vi "Number manipulating.vi"() -> ()   [LabVIEW 2017]
panel:
  in  "y 2":dbl
  in  "y":dbl
  out "x/y 2":dbl
  out "x/y":dbl
  in  "Numeric":i32
  out "Array":string[](array[string])
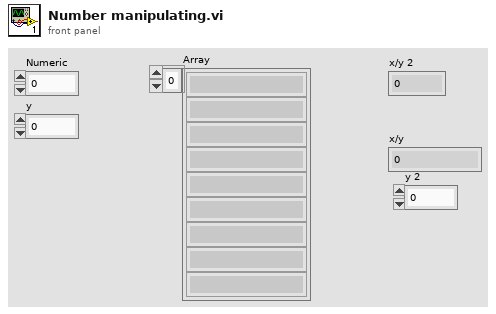
[diagram p1: front panel]
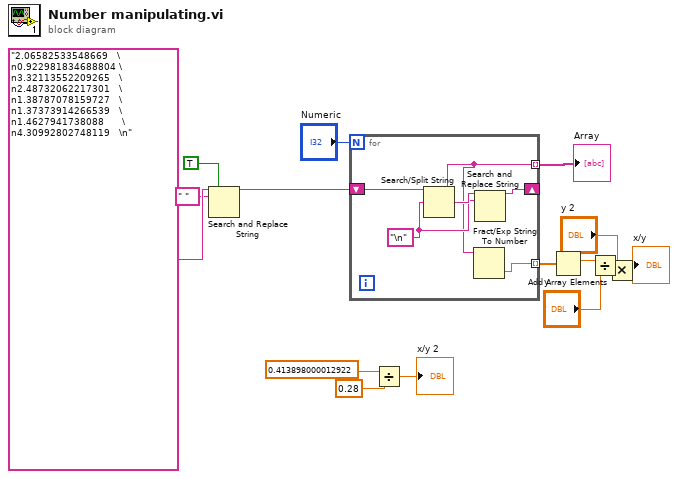
[diagram p0: block diagram]
diagram:
  n1 = Search and Replace String(replace all?=TRUE ("replace all? (F)"), input string="2.06582533548669   \n0.922981834688804 \n3.32113552209265   \n2.48732062217301   \n1.38787078159727   \n1.37373914266539   \n1.4627941738088      \n4.30992802748119   \n", search string=" ") -> (result string=w12:string)  [unwired: 5 in, 3 out]
  n2 = for {
    N: "Numeric" -> [_]
    shift-right: [w18] -> _
    shift-left: w12 -> [w21]
    tunnel: [w16] -> w11 mode=indexing
    tunnel: [w17] -> w10 mode=indexing
    w19 = "\n" ("search string")
    n3 = Search/Split String(string=w21, search string/char (-)=w19) -> (substring before match=w16:string, match + rest of string=w20:string)  [unwired: 1 in, 1 out]
    n4 = Fract/Exp String To Number(string=w16) -> (number=w17:dbl)  [unwired: 3 in, 1 out]
    n5 = Search and Replace String(input string=w20, search string=w19) -> (result string=w18:string)  [unwired: 6 in, 3 out]
  }
  "Array" <- w11
  n6 = Divide(x=0.413898000012922, y=0.28) -> (x/y=→"x/y 2":dbl)
  n7 = Add Array Elements(numeric array=w10) -> (sum=w9:dbl)
  n8 = Divide(x=w9, y="y") -> (x/y=w4:dbl)
  n9 = Multiply(x=w4, y="y 2") -> (x*y=→"x/y":dbl)
